vi "Read Test_Witness.vi"(8 "error in (no error)":errorcluster, 11 "Engine in":refnum<class "Engine.lvclass">) -> (0 "error out":errorcluster, 2 "Test_Witness":refnum<user-event>, 3 "Engine out":refnum<class "Engine.lvclass">)   [LabVIEW 2019, in "Engine.lvlib" / "Engine.lvclass"]
uses:
  Project/Engine.lvclass
  Project/Engine.lvclass/Engine.ctl
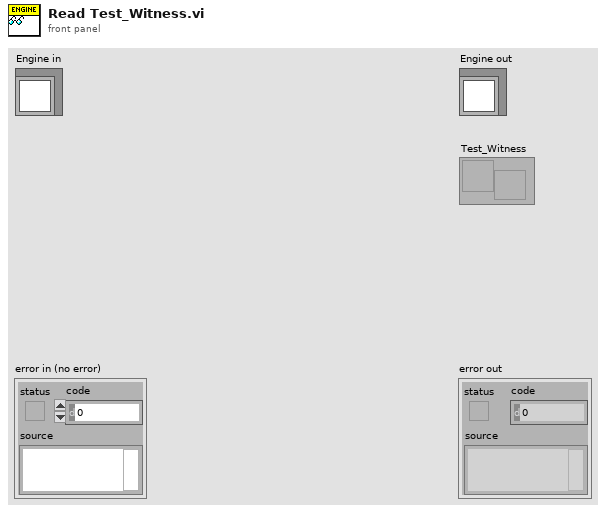
[diagram p1: front panel]
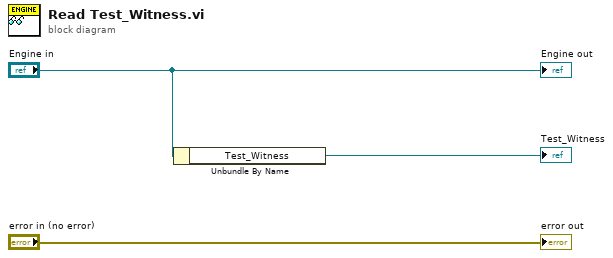
[diagram p0: block diagram]
diagram:
  n1 = Unbundle By Name("Engine in") -> ("Test_Witness"=→"Test_Witness":refnum<user-event>)
  "error out" <- "error in (no error)"
  "Engine out" <- "Engine in"
